vi "SeCrTs-Connect PPSU.vi"(8 "error In":errorcluster) -> (0 "error out":errorcluster)   [LabVIEW 2022 SP3]
panel:
  out "Data of the initialized master":string[](array[string])
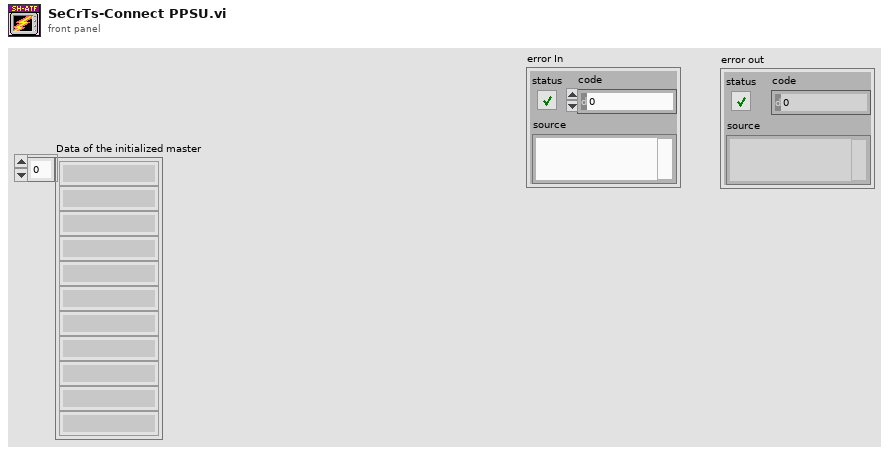
[diagram p1: front panel]
types:
  T1 = cluster{"IP range start":u8[], "IP range end":u8[], "Port":u16}
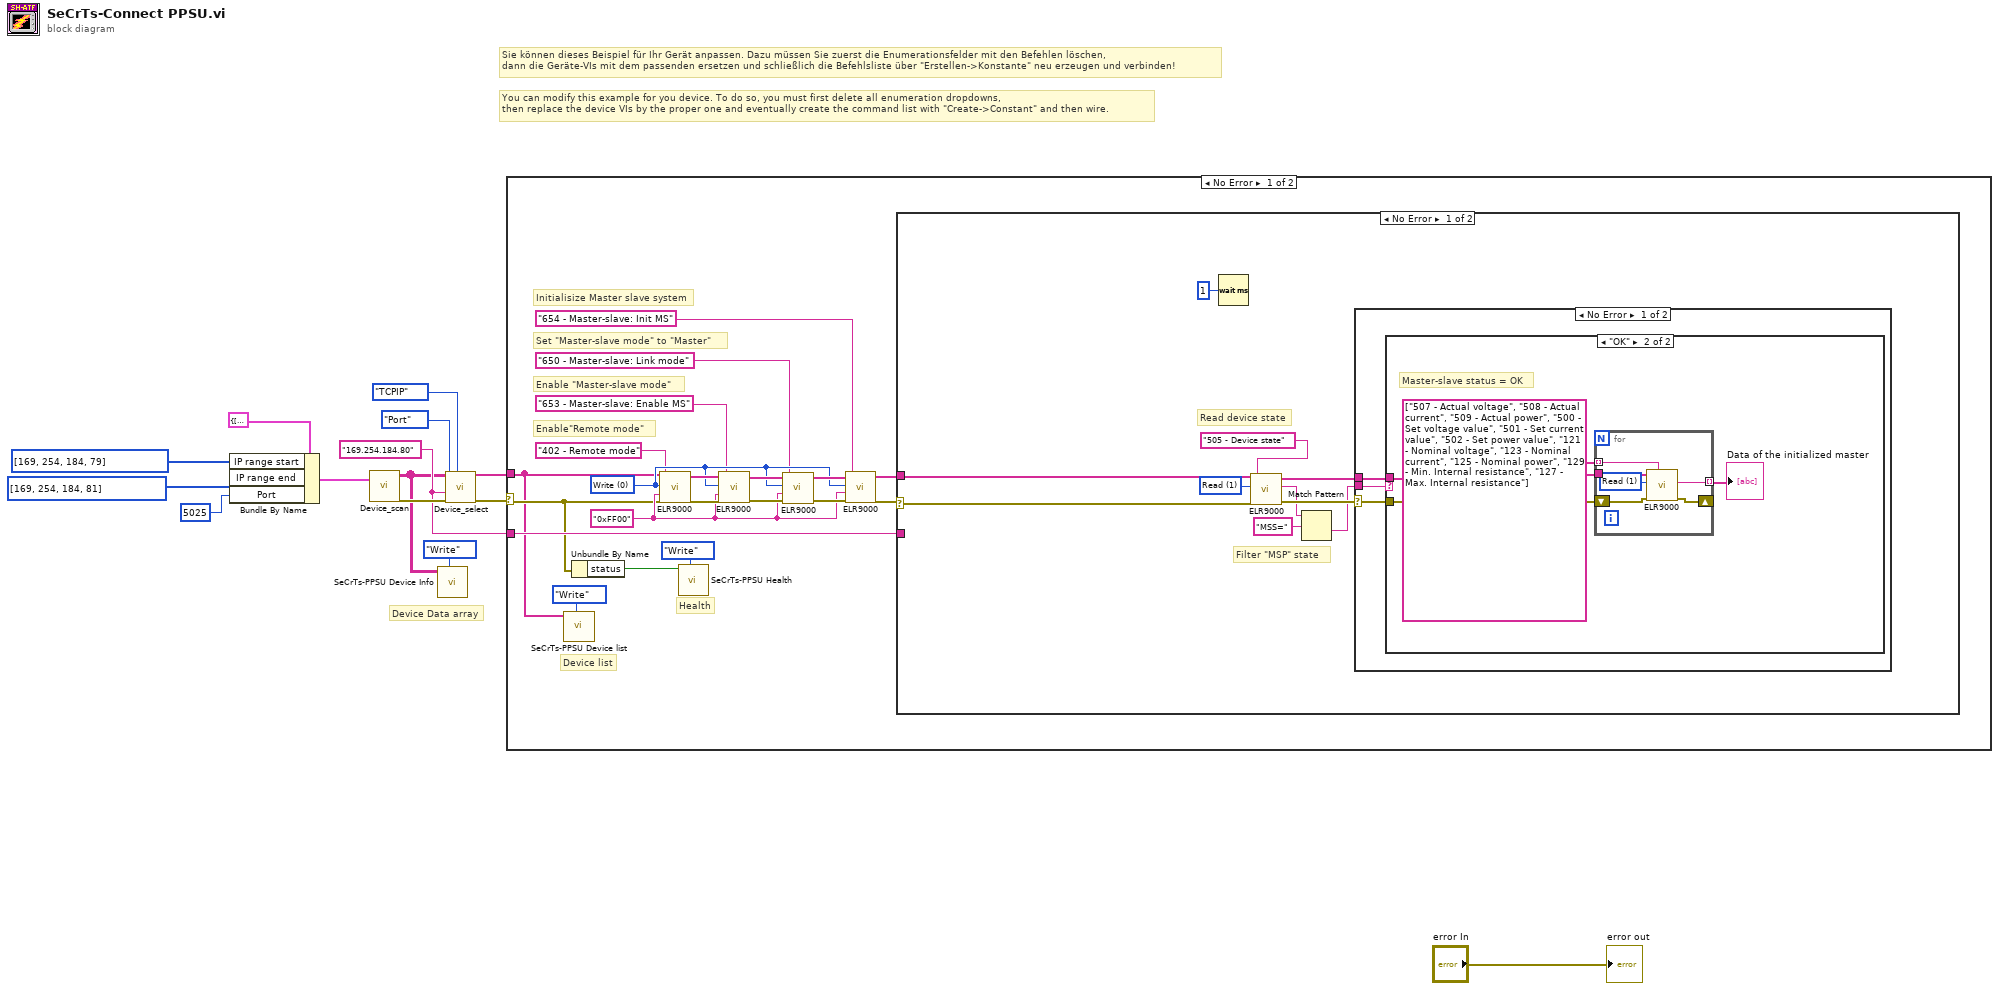
[diagram p0: block diagram]
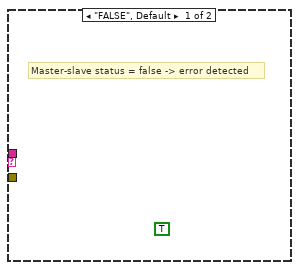
[diagram p2: hidden frame]
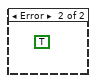
[diagram p3: hidden frame]
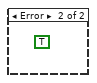
[diagram p4: hidden frame]
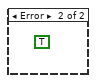
[diagram p5: hidden frame]
diagram:
  w11 = "169.254.184.80" ("Number")
  # "Device Data array"
  # "You can modify this example for you device. To do so, you must first delete all enumeration dropdowns,\nthen replace the device VIs by the proper one and eventually create the command list with \"Create->Constant\" and then wire."
  # "Sie können dieses Beispiel für Ihr Gerät anpassen. Dazu müssen Sie zuerst die Enumerationsfelder mit den Befehlen löschen,\ndann die Geräte-VIs mit dem passenden ersetzen und schließlich die Befehlsliste über \"Erstellen->Konstante\" neu erzeugen und verbinden!"
  n1 = Bundle By Name(cluster=T1 {"IP range start"=[], "IP range end"=[], "Port"=5025} ("IP settings"), "IP range start"=u8[] [169, 254, 184, 79], "IP range end"=u8[] [169, 254, 184, 81], "Port"=u16 5025) -> (w8:T1)
  n2 = call <instrlib>:"Device_scan.vi"("IP settings"=w8) -> ("Device information array"=w4:string[][], "error out"=w14:errorcluster)  [unwired: 1 in, 2 out]
  n3 = call "SeCrTs-PPSU Device Info.vi"("Enum"=enum16{"Read", "Write"}."Write", "Device information array"=w4) -> ()  [unwired: 8 in, 2 out]
  n4 = call <instrlib>:"Device_select.vi"("Reference"=enum16{"ASRL/COM", "GPIB", "TCPIP"}."TCPIP", "error in (no error)"=w14, "Alias"=w11, "Open by"=enum16{"Device Node", "Serial number", "Port"}."Port", "Device information array"=w4) -> ("error out"=w12:errorcluster, "Device information"=w13:string[])  [unwired: 2 in]
  n5 = case shown="No Error" w12 {
    selector: w12 -> [w19 _]
    tunnel: w13 -> [w15 _]
    tunnel: w11 -> [w20 _]
    frame No Error {
      w25 = u8 0 items=["Write", "Read"] ("Access")
      w26 = "0xFF00" ("Value")
      # "Health"
      # "Device list"
      # "Initialisize Master slave system"
      # "Set \"Master-slave mode\" to \"Master\""
      # "Enable \"Master-slave mode\""
      # "Enable\"Remote mode\""
      n6 = call "SeCrTs-PPSU Device list.vi"("Enum"=enum16{"Read", "Write"}."Write", "Device information array"=w15) -> ()  [unwired: 8 in, 2 out]
      n7 = Unbundle By Name(w19) -> ("status"=w17:bool)
      n8 = call <instrlib>:"ELR9000.vi"("Command list"="402 - Remote mode", "Error in"=w19, "Value"=w26, "Access"=w25, "Device information in"=w15) -> ("Error out"=w32:errorcluster, "Device information out"=w31:string[])  [unwired: 1 in, 2 out]
      n9 = call "SeCrTs-PPSU Health.vi"("Enum"=enum16{"Read", "Write"}."Write", "ppsu health"=w17) -> ()  [unwired: 8 in, 2 out]
      n10 = call <instrlib>:"ELR9000.vi"("Command list"="653 - Master-slave: Enable MS", "Error in"=w32, "Value"=w26, "Access"=w25, "Device information in"=w31) -> ("Error out"=w30:errorcluster, "Device information out"=w27:string[])  [unwired: 1 in, 2 out]
      n11 = call <instrlib>:"ELR9000.vi"("Command list"="650 - Master-slave: Link mode", "Error in"=w30, "Value"=w26, "Access"=w25, "Device information in"=w27) -> ("Error out"=w29:errorcluster, "Device information out"=w28:string[])  [unwired: 1 in, 2 out]
      n12 = call <instrlib>:"ELR9000.vi"("Command list"="654 - Master-slave: Init MS", "Error in"=w29, "Value"=w26, "Access"=w25, "Device information in"=w28) -> ("Error out"=w34:errorcluster, "Device information out"=w33:string[])  [unwired: 1 in, 2 out]
      n13 = case shown="No Error" w34 {
        selector: w34 -> [w43 _]
        tunnel: w33 -> [w44 _]
        tunnel: w20 -> [_ _]
        frame No Error {
          w42 = u8 1 items=["Write", "Read"] ("Access")
          # "Read device state"
          # "Filter \"MSP\" state"
          n14 = Wait (ms)(milliseconds to wait=u32 1 ("Zu wartende ms")) -> ()  [unwired: 1 out]
          n15 = call <instrlib>:"ELR9000.vi"("Command list"="505 - Device state", "Error in"=w43, "Access"=w42, "Device information in"=w44) -> ("Error out"=w41:errorcluster, "Read data"=w39:string, "Device information out"=w40:string[])  [unwired: 2 in, 1 out]
          n16 = Match Pattern(string=w39, regular expression="MSS=" ("regulärer Ausdruck")) -> (after substring=w37:string)  [unwired: 1 in, 3 out]
          n17 = case shown="No Error" w41 {
            selector: w41 -> [w45 _]
            tunnel: w37 -> [w47 _]
            tunnel: w40 -> [w46 _]
            frame No Error {
              n18 = case shown="\"OK\"" w47 {
                tunnel: w46 -> [_ w50]
                tunnel: w45 -> [_ w49]
                frame "FALSE", Default {
                  (unwired) TRUE
                  # "Master-slave status = false -> error detected"
                }
                frame "OK" {
                  # "Master-slave status = OK"
                  n19 = for {
                    tunnel: w50 -> [w57]
                    tunnel: string[] ["507 - Actual voltage", "508 - Actual current", "509 - Actual power", "500 - Set voltage value", "501 - Set current value", "502 - Set power value", "121 - Nominal voltage", "123 - Nominal current", "125 - Nominal power", "129 - Min. Internal resistance", "127 - Max. Internal resistance"] -> [w55] mode=indexing
                    shift-right: [w53] -> _
                    shift-left: w49 -> [w54]
                    tunnel: [w52] -> w51 mode=indexing
                    w56 = u8 1 items=["Write", "Read"] ("Access")
                    n20 = call <instrlib>:"ELR9000.vi"("Command list"=w55, "Error in"=w54, "Access"=w56, "Device information in"=w57) -> ("Error out"=w53:errorcluster, "Read data"=w52:string)  [unwired: 2 in, 2 out]
                  }
                  "Data of the initialized master" <- w51
                }
              }
            }
            frame Error {
              (unwired) TRUE
            }
          }
        }
        frame Error {
          (unwired) TRUE
        }
      }
    }
    frame Error {
      (unwired) TRUE
    }
  }
  "error out" <- "error In"
